vi "Initialize.vi"(8 "error in (no error)":errorcluster, 11 "VISA resource name":refnum<visa-resource-name>="TCPIP::127.0.0.1::8888::SOCKET") -> (0 "error out":errorcluster, 2 "ID result":string, 3 "VISA resource name out":refnum<visa-resource-name>)   [LabVIEW 2023, in "Thermotron 8800.lvlib"]
doc: "Establishes communication with the instrument and optionally performs an instrument identification query and/or an instrument reset. It also places the instrument in a default state needed for other instrument driver operations. Therefore, call this VI before calling other instrument driver VIs for this instrument. Generally, you need to call the <b>Initialize</b> VI only once at the beginning of an application."
uses:
  Thermotron 8800.lvlib
  <vilib>/Instr/_visa.llb/VISA Configure Serial Port (Instr).vi
panel:
  in  "ID Query":bool=TRUE
  in  "Serial Configuration":T1={"Baud Rate"=19200, "Parity"=0, "Data Bits"=8, "Stop Bits"=10, "Flow Control"=0} {"Flow Control" items=["None", "XON/XOFF", "RTS/CTS", "XON/XOFF & RTS/CTS", "DTR/DSR", "XON/XOFF & DTR/DSR"]; "Stop Bits" items=["1.0"=10, "1.5"=15, "2.0"=20]; "Data Bits" items=["7"=7, "8"=8]; "Parity" items=["None", "Odd", "Even", "Mark", "Space"]; "Baud Rate" items=["300"=300, "600"=600, "1200"=1200, "2400"=2400, "4800"=4800, "9600"=9600, "19200"=19200]}
  # "(c) 2017 Thermotron Industries.  ALL RIGHTS RESERVED."
  # "GPIB Configuration\nRequirements: NI-488.2 and NI-VISA Drivers\nInstructions:\n1. Ensure the resource specified in the VISA GPIB Resource control is properly configured in NI Measurement & Automation Explorer.\n(Devices and Interfaces, GPIB0, Properties = Use defaults except for Termination Settings:\n    Send EOI at End of Write\n    Terminate Read on EOS\n    EOS Byte = 13\n    8-bit EOS compare\n    Set EOI with EOS on Write)\n2. Chamber controller computer I/O GPIB setup:\n    Send EOI = yes\n    Terminator = Last Input\n    Send Acknowledgement = yes"
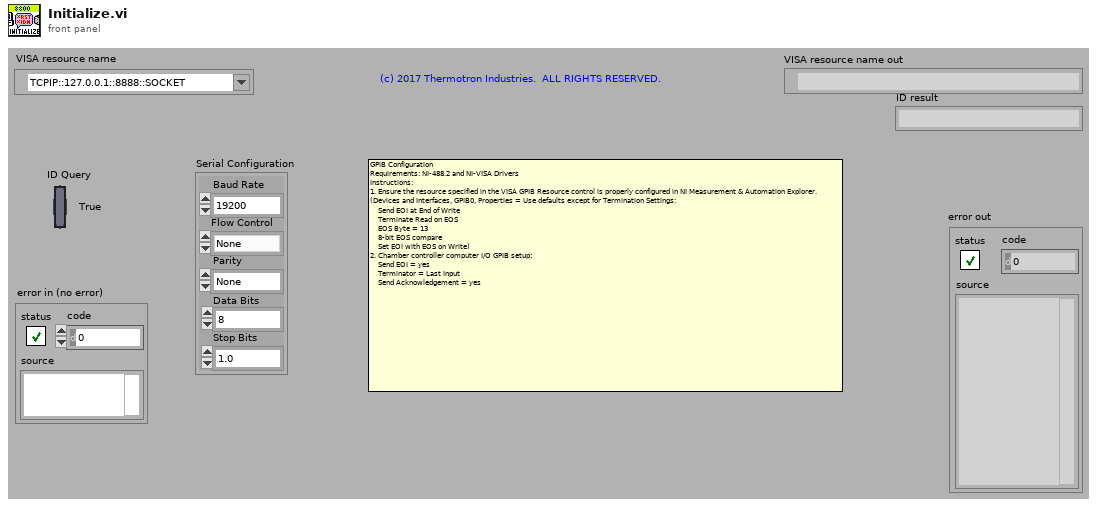
[diagram p1: front panel]
types:
  T1 = cluster{"Baud Rate":u32, "Parity":u16, "Data Bits":u16, "Stop Bits":u16, "Flow Control":u16}
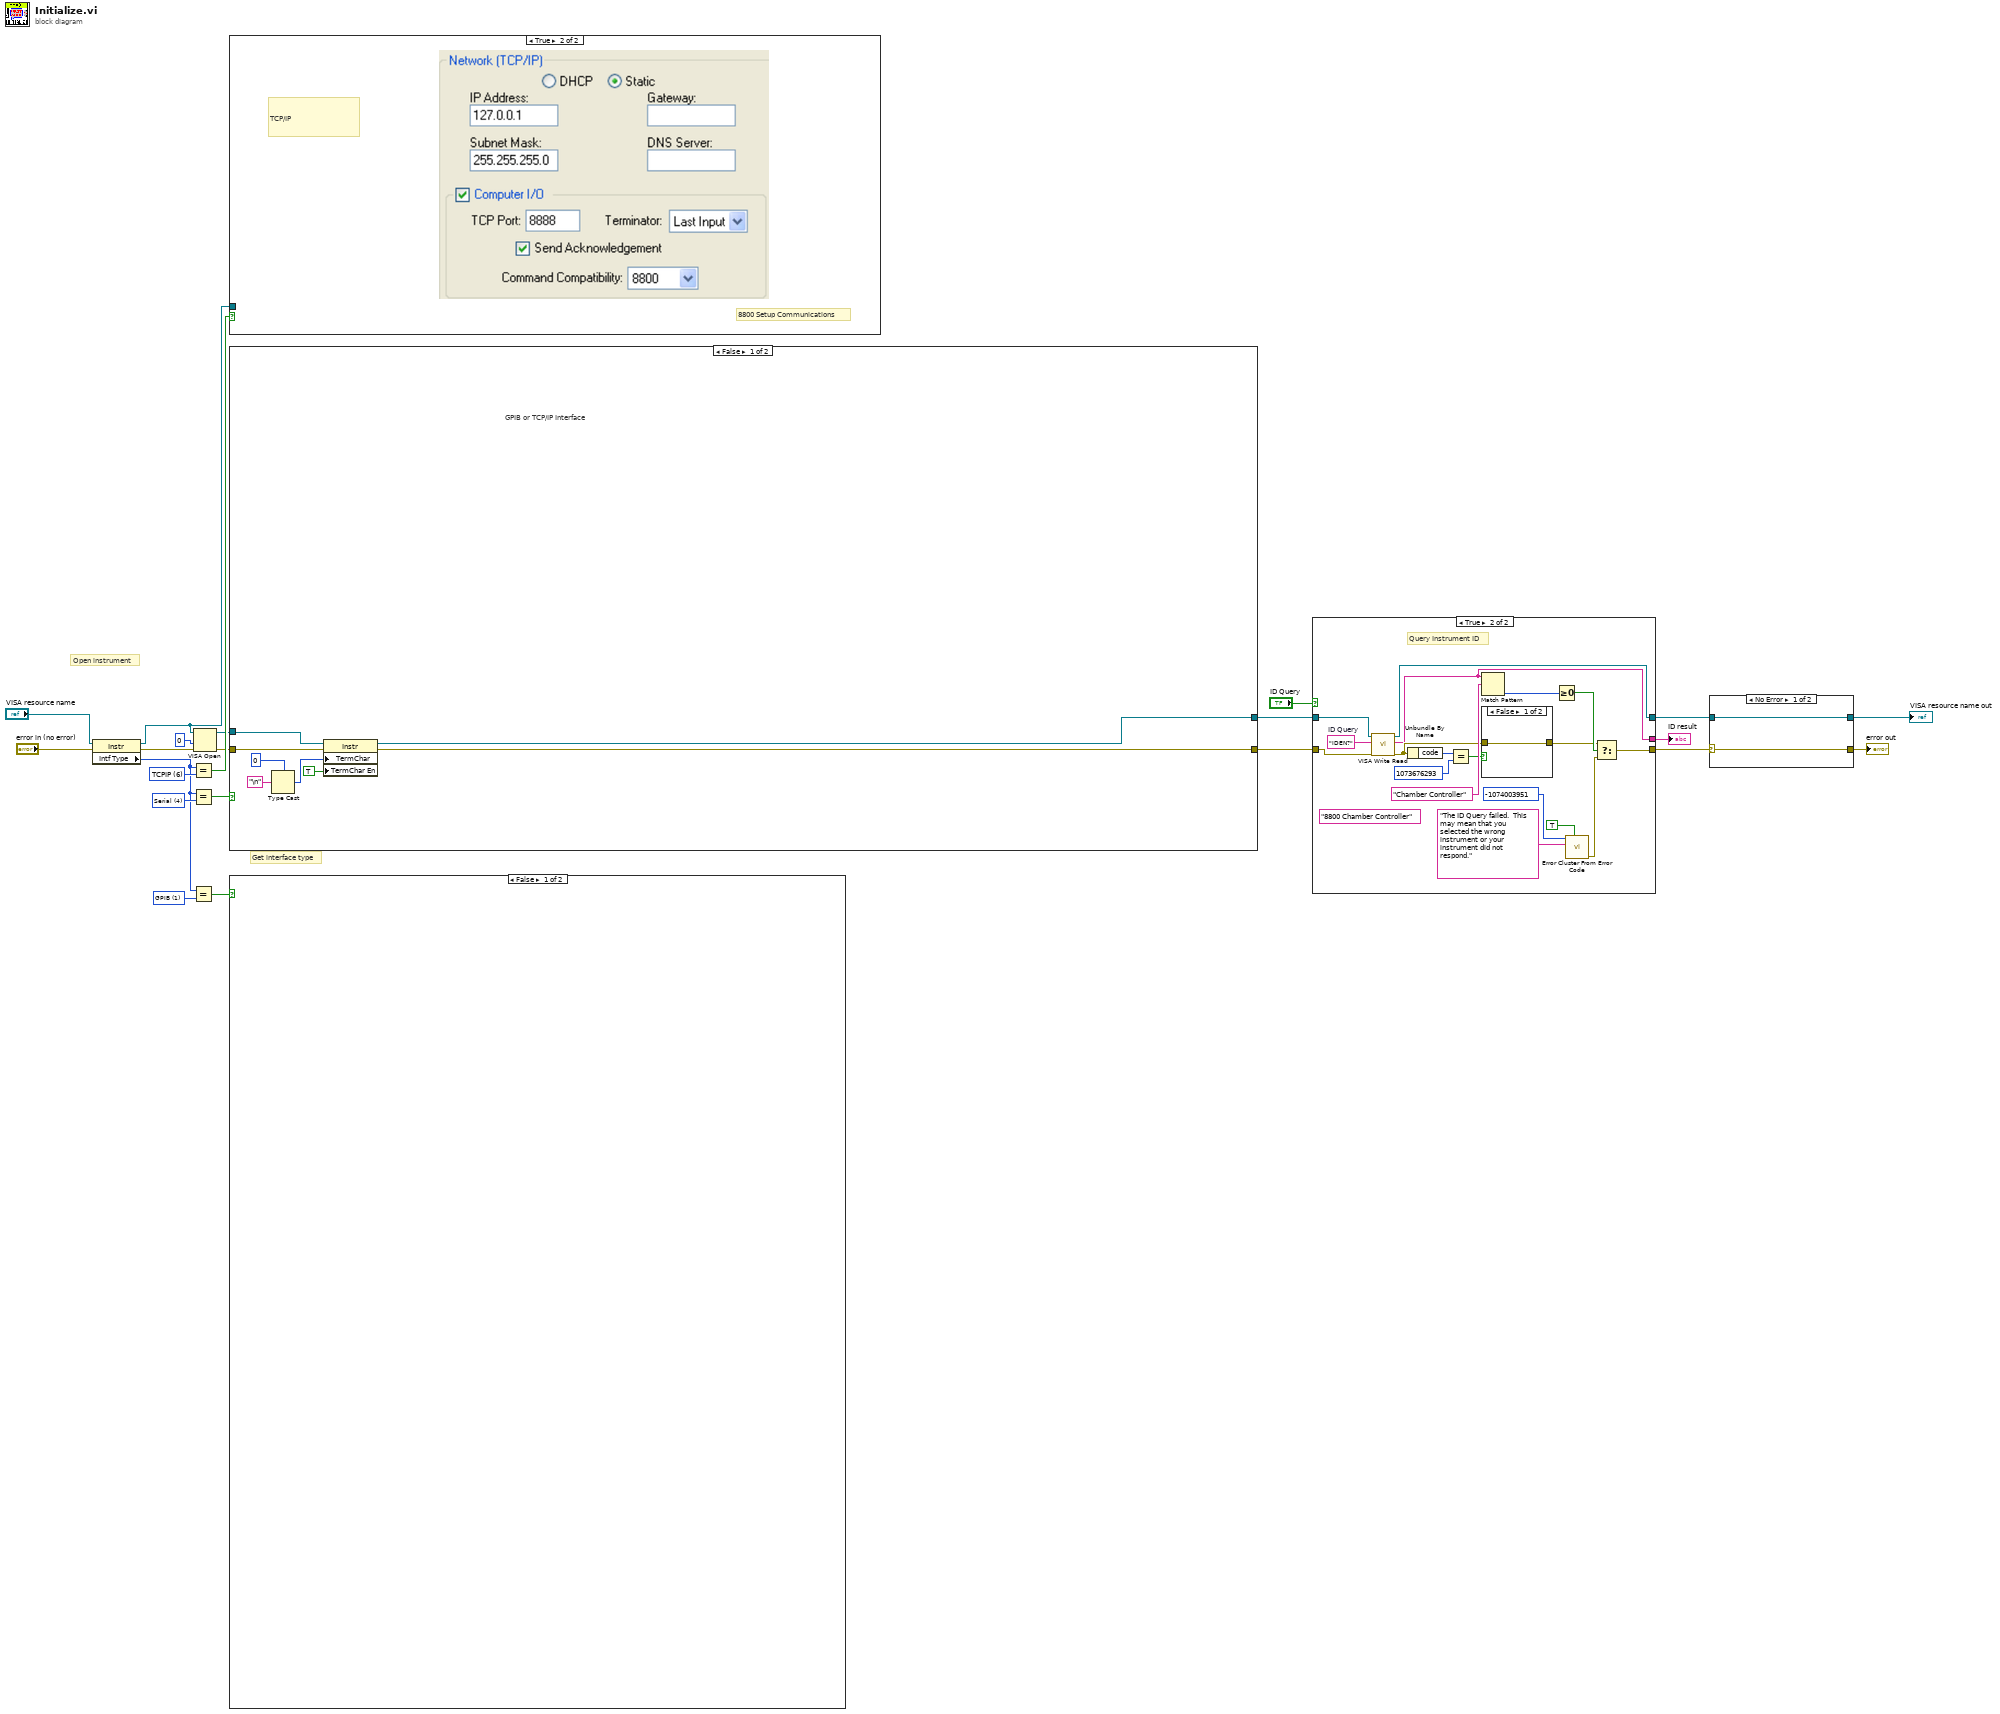
[diagram p0: block diagram]
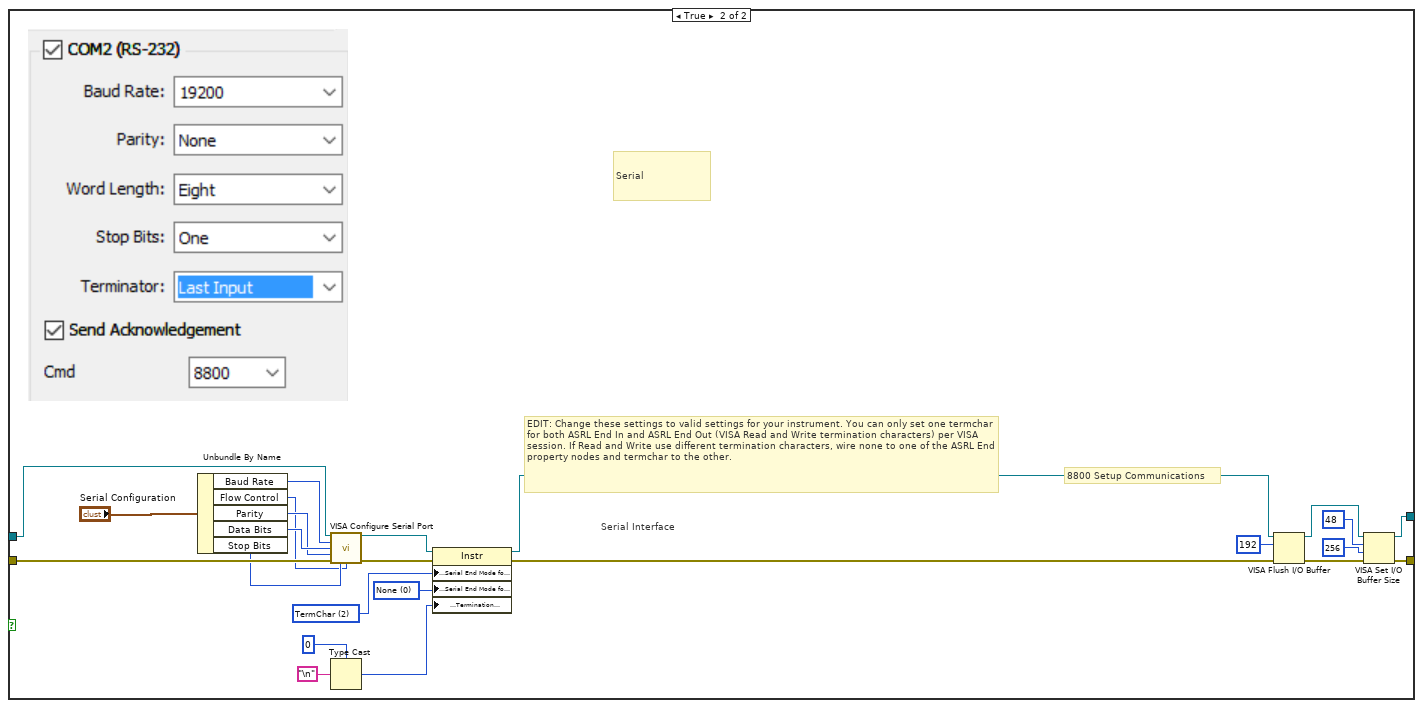
[diagram p4: hidden frame]
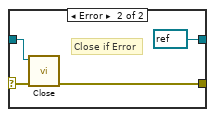
[diagram p5: hidden frame]
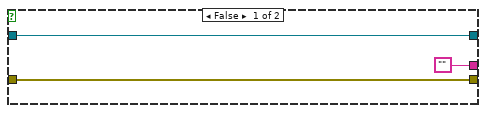
[diagram p6: hidden frame]
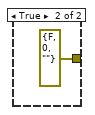
[diagram p7: hidden frame]
diagram:
  w8 = u16 1 items=["GPIB"=1, "VXI"=2, "GPIB-VXI"=3, "Serial"=4, "PXI"=5, "TCPIP"=6, "USB"=7] ("Interface Information:Interface Type")
  w21 = u16 6 items=["GPIB"=1, "VXI"=2, "GPIB-VXI"=3, "Serial"=4, "PXI"=5, "TCPIP"=6, "USB"=7] ("Interface Information:Interface Type")
  w15 = u16 4 items=["GPIB"=1, "VXI"=2, "GPIB-VXI"=3, "Serial"=4, "PXI"=5, "TCPIP"=6, "USB"=7] ("Interface Information:Interface Type")
  # "Get interface type"
  # "Open instrument"
  n1 = property class="Instr"(reference="VISA resource name", error in="error in (no error)") -> (reference out=w2:refnum<visa-resource-name>, error out=w1:errorcluster, "Intf Type"=w5:u16)
  n2 = Equal?(x=w5, y=w21) -> (x = y?=w22:bool)
  n3 = Equal?(x=w5, y=w15) -> (x = y?=w14:bool)
  n4 = Equal?(x=w5, y=w8) -> (x = y?=w7:bool)
  n5 = VISA Open(access mode=u32 0, error in (no error)=w1, VISA resource name=w2) -> (VISA resource name=w17:refnum<visa-resource-name>, error out=w18:errorcluster)  [unwired: 2 in]
  n6 = case shown="True" w22 {
    tunnel: w2 -> [_ _]
    frame False {
    }
    frame True {
      # "TCP/IP"
      # "8800 Setup Communications"
    }
  }
  n7 = case shown="False" w14 {
    tunnel: [w28 w44] -> w12
    tunnel: [w27 w43] -> w13
    tunnel: w17 -> [w30 w53]
    tunnel: w18 -> [w29 w49]
    frame False {
      # "GPIB or TCP/IP Interface"
      n8 = Type Cast(type=u8 0, x="\n") -> (*(type *) &x=w24:u8)
      n9 = property class="Instr"(reference=w30, error in=w29, "TermChar"=w24, "TermChar En"=TRUE ("Message Based Settings:Termination Character Enable")) -> (reference out=w28:refnum<visa-resource-name>, error out=w27:errorcluster)
    }
    frame True {
      w40 = u16 0 items=["None", "Last Bit", "TermChar", "Break"] ("Serial Settings:End Mode for Writes")
      w42 = u16 2 items=["None", "LastBit", "TermChar"] ("Serial Settings:Serial End Mode for Reads")
      # "Serial"
      # "8800 Setup Communications"
      # "Serial Interface"
      # "EDIT: Change these settings to valid settings for your instrument. You can only set one termchar for both ASRL End In and ASRL End Out (VISA Read and Write termination characters) per VISA session. If Read and Write use different termination characters, wire none to one of the ASRL End property nodes and termchar to the other."
      n10 = Unbundle By Name("Serial Configuration") -> ("Baud Rate"=w52:u32, "Flow Control"=w47:u16, "Parity"=w50:u16, "Data Bits"=w51:u16, "Stop Bits"=w48:u16)
      n11 = call-poly "VISA Configure Serial Port"("VISA resource name"=w53, "baud rate (9600)"=w52, "data bits (8)"=w51, "parity (0:none)"=w50, "error in (no error)"=w49, "stop bits (10: 1 bit)"=w48, "flow control (0:none)"=w47) -> ("VISA resource name out"=w45:refnum<visa-resource-name>, "error out"=w46:errorcluster)  [unwired: 7 in]
      n12 = Type Cast(type=u8 0, x="\n") -> (*(type *) &x=w38:u8)
      n13 = property class="Instr"(reference=w45, error in=w46, "Serial Settings:Serial End Mode for Reads"=w42, "Serial Settings:Serial End Mode for Writes"=w40, "Message Based Settings:Termination Character"=w38) -> (reference out=w35:refnum<visa-resource-name>, error out=w36:errorcluster)
      n14 = VISA Flush I/O Buffer(VISA resource name=w35, mask (16)=u16 192, error in (no error)=w36) -> (VISA resource name out=w31:refnum<visa-resource-name>, error out=w32:errorcluster)
      n15 = VISA Set I/O Buffer Size(VISA resource name=w31, mask (16)=u16 48, size (4096)=u32 256 ("size (0)"), error in (no error)=w32) -> (VISA resource name out=w44:refnum<visa-resource-name>, error out=w43:errorcluster)
    }
  }
  n16 = case shown="False" w7 {
    frame False {
    }
    frame True {
      # "NI MAX GPIB0 settings"
      # "8800 Setup Communications"
      # "Overview: Demonstrates the use of the VISA functions to communicate to a GPIB instrument.\nRequirements: NI-488.2 and NI-VISA Drivers\nInstructions:\n1. Ensure the resource specified in the VISA GPIB Resource control is properly configured in NI Measurement & Automation Explorer.\n(Devices and Interfaces, GPIB0, Properties = Use defaults except for Termination Settings: Send EOI at End of Write, Terminate Read on EOS, EOS Byte = 13, 8-bit EOS compare, Set EOI with EOS on Write)\n2. Chamber controller computer I/O GPIB setup: Send EOI = yes, Terminator = CR, Send Ack = yes\n3. Run the VI."
    }
  }
  n17 = case shown="True" "ID Query" {
    tunnel: [w56 w75] -> w10
    tunnel: [w57 w59] -> w9
    tunnel: w12 -> [w57 w63]
    tunnel: w13 -> [w56 w61]
    tunnel: ["" w58] -> w6
    frame False {
    }
    frame True {
      (unwired) "8800 Chamber Controller"
      w62 = "IDEN?"  # ID Query
      # "Query Instrument ID"
      n18 = call "VISA Write Read.vi"("error in (no error)"=w61, "8800 Command"=w62, "VISA Refnum in"=w63) -> ("error out"=w60:errorcluster, "read buffer"=w58:string, "VISA Refnum out"=w59:refnum<visa-resource-name>)  [unwired: 6 in]
      n19 = Unbundle By Name(w60) -> ("code"=w67:i32)
      n20 = Equal?(x=w67, y=1073676293) -> (x = y?=w65:bool)
      n21 = Match Pattern(string=w58, regular expression="Chamber Controller") -> (offset past match=w69:i32)  [unwired: 1 in, 3 out]
      n22 = case shown="False" w65 {
        tunnel: w60 -> [w76 _]
        tunnel: [w76 errorcluster {"status"=FALSE, "code"=0, "source"=""} ("error out")] -> w64
        frame False {
        }
        frame True {
        }
      }
      n23 = Greater Or Equal To 0?(x=w69) -> (x >= 0?=w68:bool)
      n24 = call <vilib>:"Error Cluster From Error Code.vi"("show call chain? (False)"=TRUE, "error message (\"\")"="The ID Query failed.  This may mean that you selected the wrong instrument or your instrument did not respond." ("Source (VI Name)"), "error code (0)"=-1074003951 ("Code")) -> ("error out"=w73:errorcluster)  [unwired: 6 in]
      n25 = Select(t=w64, s=w68, f=w73) -> (s? t:f=w75:errorcluster)
    }
  }
  "ID result" <- w6
  n26 = case shown="No Error" w10 {
    selector: w10 -> [w78 w81]
    tunnel: w9 -> [w79 w82]
    tunnel: [w79 refnum<visa-resource-name> refnum ("VISA resource name out")] -> w19
    tunnel: [w78 w83] -> w20
    frame No Error {
    }
    frame Error {
      # "Close if Error"
      n27 = call "Close.vi"("error in (no error)"=w81, "VISA resource name"=w82) -> ("error out"=w83:errorcluster)  [unwired: 9 in]
    }
  }
  "VISA resource name out" <- w19
  "error out" <- w20
